vi "DTMF.vi"() -> ()   [LabVIEW 2014]
uses:
  <vilib>/sound2/lvsound2.llb/Sampling Mode.ctl
  <vilib>/sound2/lvsound2.llb/Sound Data Format.ctl
  <vilib>/sound2/lvsound2.llb/Sound Input Read (DBL).vi
  <vilib>/measure/maspectr.llb/FFT Power Spectrum and PSD for N Chan.vi
  <vilib>/measure/NI_MAPro.lvlib
panel:
  in  "Tab Control":enum32{"Info.", "Output", "Details"}(tab)
  in  "Stop":bool
  out "Dialed Number":string
  in  "Number of Samples/ch":i32=5000
  in  "Device ID":u32 format="%.0x"
  out "Raw Data":waveform(dbl)[](graph)
  out "FFT":cluster{"f0":dbl, "df":dbl, "magnitude":dbl[]}[](graph)
  out "Power Spectrum / PSD":cluster{"f0":dbl, "df":dbl, "magnitude":dbl[]}[](array[cluster]) {"magnitude" format="%.2p"; "f0" format="%.2p"; "df" format="%.2p"}
  out "f0":dbl
  out "df":dbl
  out "magnitude":dbl[](array[numeric])
  out "output array":dbl[](array[numeric])
  out "Max":dbl
  out "Coloumn":u32
  out "Raw":u32
  out "Min":dbl
  out "concatenated string":string
  # "This programthe can detect DTMF type sounds and decode them to digits as you know every digits in DTMF modulation contain two tone signal with specified frequency.\nfirst program captures sound from environment and make FFT from that , then the created PSD array processed to retrieve first 2frequency with most power and then realize reffered digit."
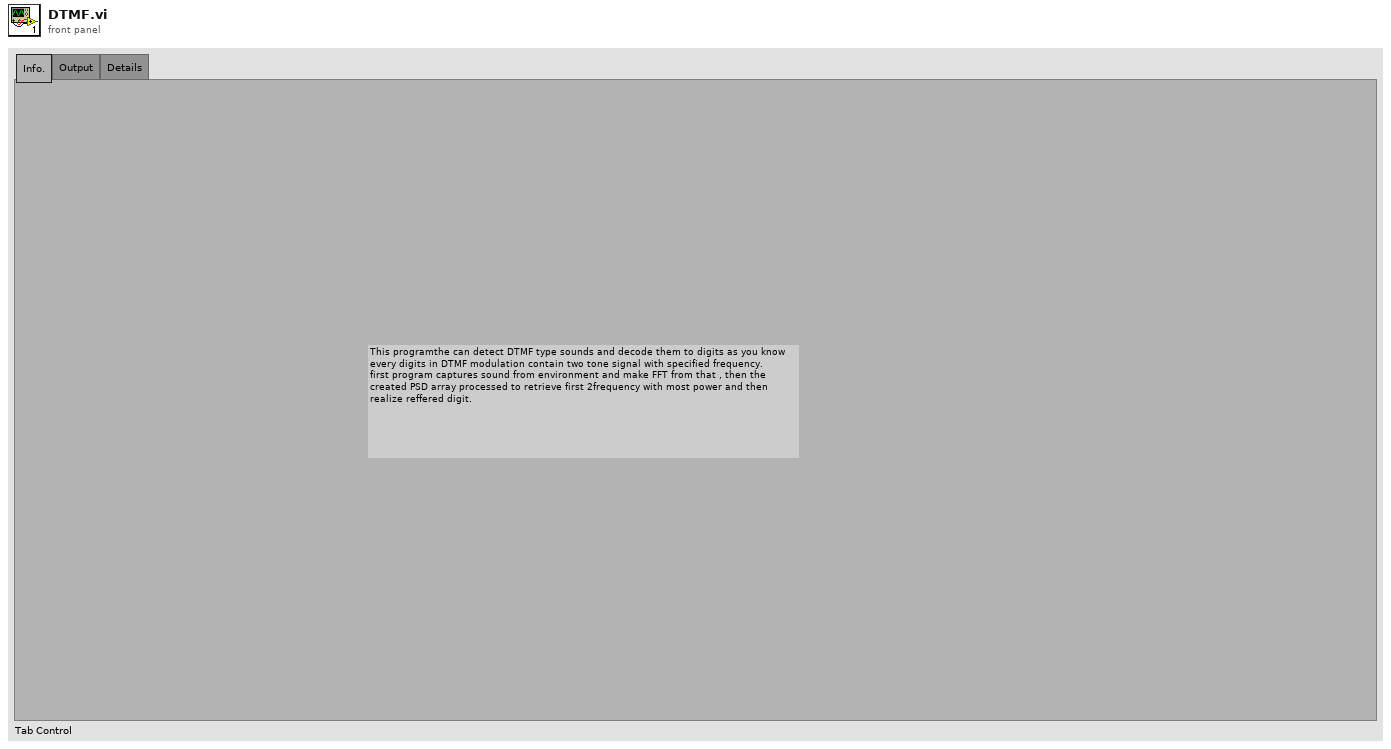
[diagram p1: front panel]
types:
  T1 = typedef "Sound Data Format.ctl" = cluster{"sample rate (S/s)":dbl, "number of channels":i32, "bits per sample":i32}
  T2 = typedef "Sampling Mode.ctl" = i32
  T3 = typedef "Sound Input Task ID.ctl" = u32
  T4 = cluster{"Power Spectrum / PSD[0]":cluster{"f0":dbl, "df":dbl, "magnitude":dbl[]}, "Power Spectrum / PSD[1]":cluster{"f0":dbl, "df":dbl, "magnitude":dbl[]}, "Power Spectrum / PSD[2]":cluster{"f0":dbl, "df":dbl, "magnitude":dbl[]}, "Power Spectrum / PSD[3]":cluster{"f0":dbl, "df":dbl, "magnitude":dbl[]}, "Power Spectrum / PSD[4]":cluster{"f0":dbl, "df":dbl, "magnitude":dbl[]}, "Power Spectrum / PSD[5]":cluster{"f0":dbl, "df":dbl, "magnitude":dbl[]}, "Power Spectrum / PSD[6]":cluster{"f0":dbl, "df":dbl, "magnitude":dbl[]}, "Power Spectrum / PSD[7]":cluster{"f0":dbl, "df":dbl, "magnitude":dbl[]}, "Power Spectrum / PSD[8]":cluster{"f0":dbl, "df":dbl, "magnitude":dbl[]}}
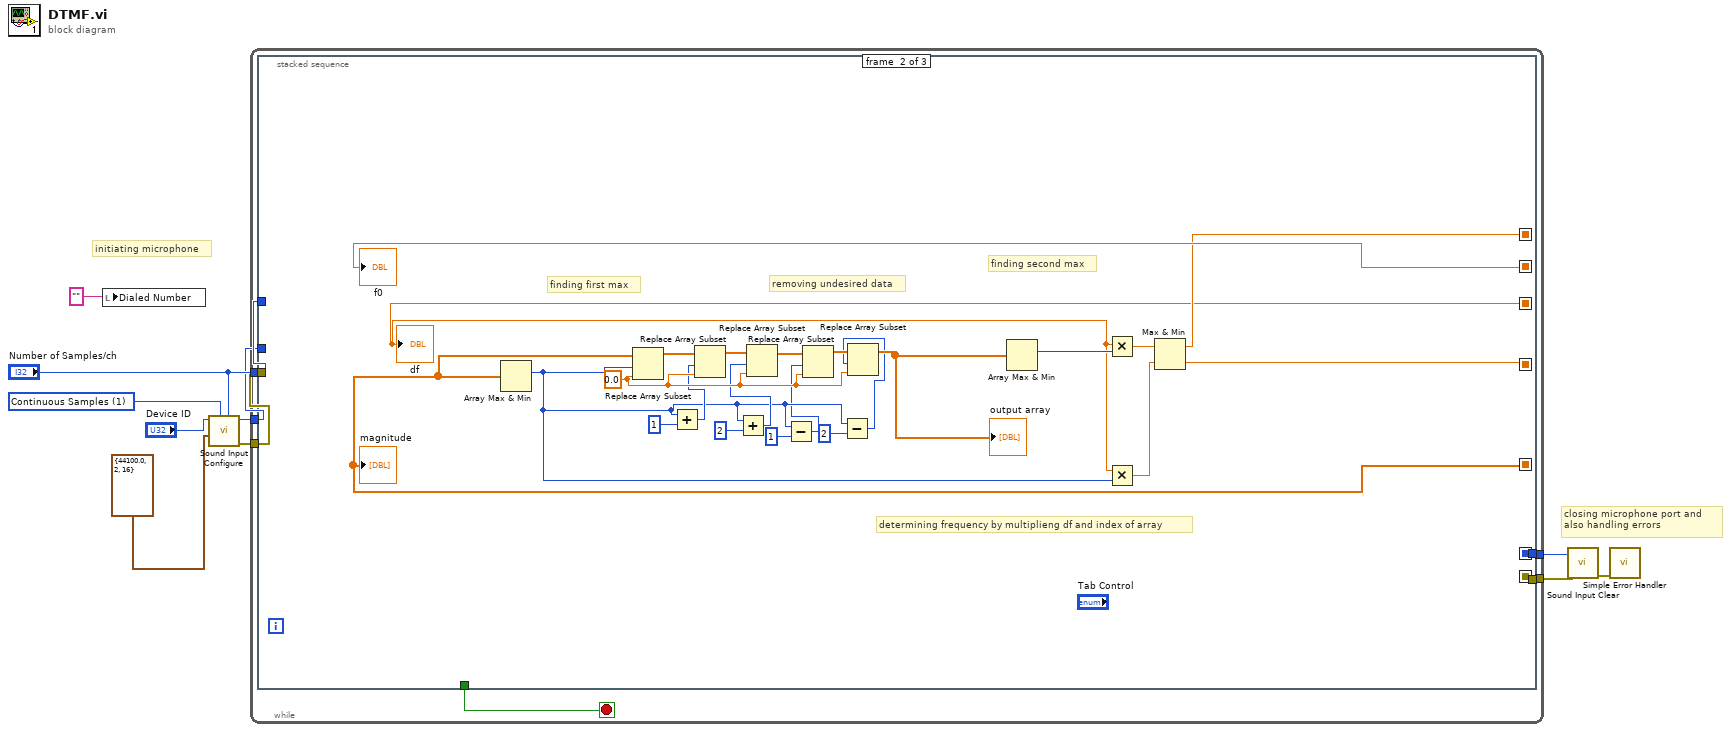
[diagram p0: block diagram]
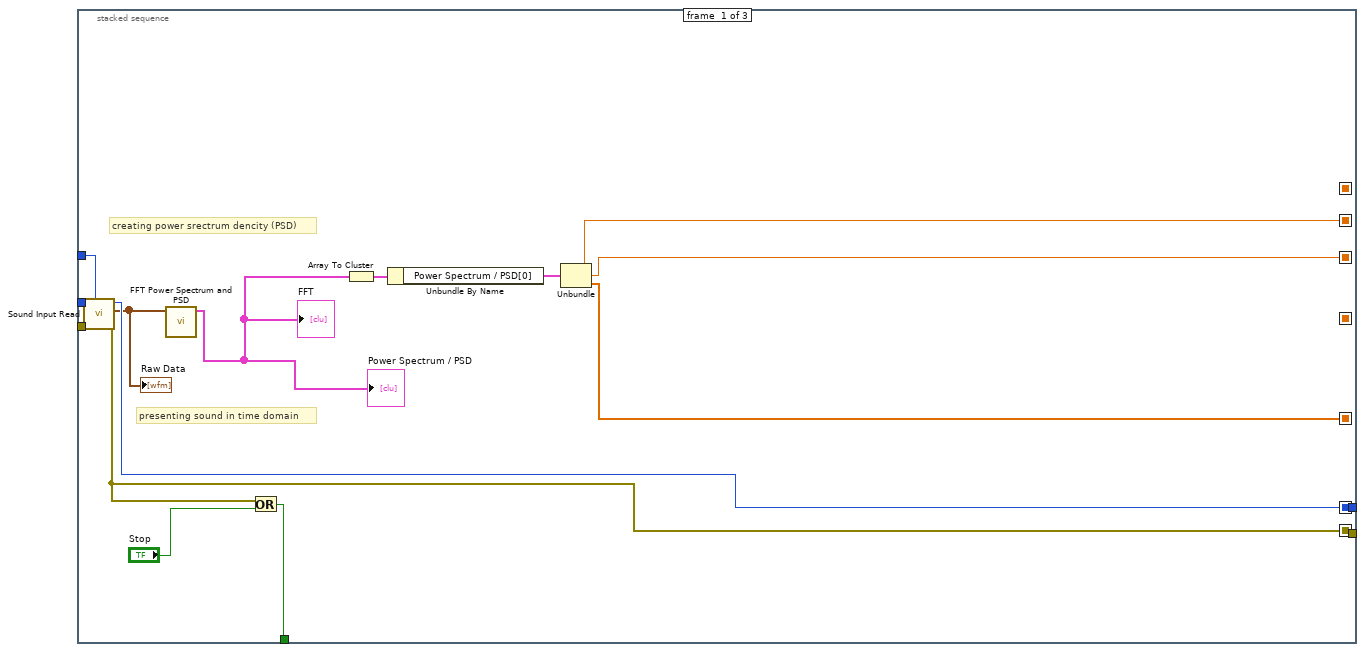
[diagram p2: hidden frame]
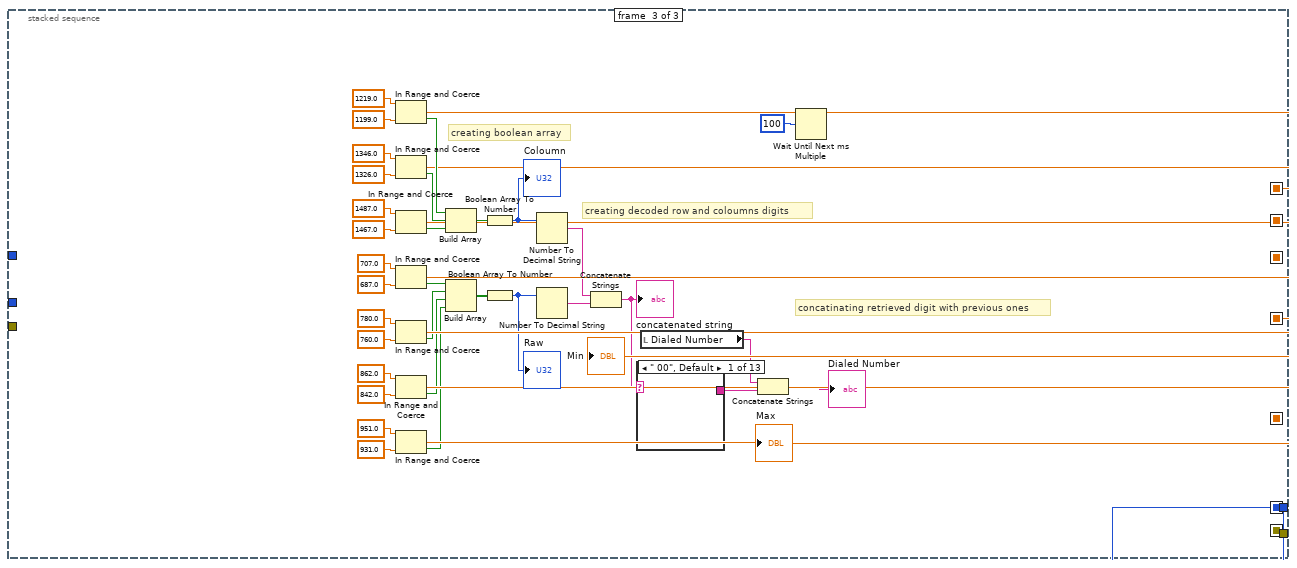
[diagram p3: hidden frame]
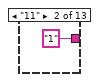
[diagram p4: hidden frame]
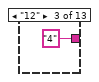
[diagram p5: hidden frame]
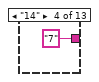
[diagram p6: hidden frame]
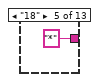
[diagram p7: hidden frame]
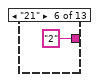
[diagram p8: hidden frame]
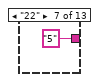
[diagram p9: hidden frame]
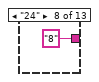
[diagram p10: hidden frame]
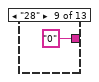
[diagram p11: hidden frame]
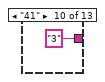
[diagram p12: hidden frame]
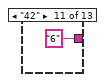
[diagram p13: hidden frame]
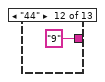
[diagram p14: hidden frame]
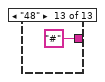
[diagram p15: hidden frame]
diagram:
  w9 = T2 1 items=["Finite Samples", "Continuous Samples"] ("sample mode")
  # "closing microphone port and \nalso handling errors"
  # "initiating microphone"
  n1 = local write "Dialed Number"("") -> ()
  n2 = call <vilib>:"Sound Input Configure.vi"("number of samples/ch"="Number of Samples/ch", "sample mode"=w9, "sound format"=T1 {"sample rate (S/s)"=44100.0, "number of channels"=2, "bits per sample"=16} ("Sound Format"), "device ID"="Device ID") -> ("error out"=w5:errorcluster, "task ID"=w6:T3)  [unwired: 6 in]
  n3 = while {
    tunnel: "Number of Samples/ch" -> [w16]
    tunnel: [w15] -> w1
    tunnel: [w14] -> w2
    tunnel: w6 -> [w13]
    tunnel: w5 -> [w12]
    stop <- w11 stop-if-true
    n4 = stacked-sequence {
      seq-local: [w29 _ _] -> [_ w55 _]
      seq-local: [w28 _ _] -> [_ w54 _]
      seq-local: [w20 _ _] -> [_ w47 _]
      seq-local: [w21 _ _] -> [_ w50 _]
      seq-local: [w19 _ _] -> [_ w31 _]
      seq-local: [_ w55 _] -> [_ _ w91]
      seq-local: [_ w54 _] -> [_ _ w90]
      seq-local: [_ w49 _] -> [_ _ w80]
      seq-local: [_ w48 _] -> [_ _ w78]
      tunnel: w16 -> [w30 _ _]
      tunnel: w13 -> [w27 _ _]
      tunnel: w12 -> [w26 _ _]
      tunnel: [w17 _ _] -> w11
      tunnel: [_ _ w91] -> w15
      tunnel: [_ _ w90] -> w14
      frame #0 {
        # "presenting sound in time domain"
        # "creating power srectrum dencity (PSD)"
        n5 = call-poly <vilib>:"Sound Input Read.vi"("number of samples/ch"=w30, "error in (no error)"=w26, "task ID"=w27) -> ("error out"=w29:errorcluster, "data"=w23:waveform(dbl)[], "task ID out"=w28:T3)  [unwired: 6 in]
        "Raw Data" <- w23
        n6 = call-poly <vilib>:"FFT Power Spectrum and PSD.vi"("time signals"=w23) -> ("Power Spectrum / PSD"=w22:cluster{"f0":dbl, "df":dbl, "magnitude":dbl[]}[])  [unwired: 7 in, 3 out]
        "FFT" <- w22
        "Power Spectrum / PSD" <- w22
        n7 = Or(x=w29, y="Stop") -> (x .or. y?=w17:bool)
        n8 = Array To Cluster(array=w22) -> (cluster=w25:T4)
        n9 = Unbundle By Name(w25) -> ("Power Spectrum / PSD[0]"=w24:cluster{"f0":dbl, "df":dbl, "magnitude":dbl[]})
        n10 = Unbundle(w24) -> ("f0"=w21:dbl, "df"=w20:dbl, "magnitude"=w19:dbl[])
      }
      frame #1 {
        w41 = 0.0 ("new element/subarray")
        # "removing undesired data"
        # "determining frequency by multiplieng df and index of array"
        # "finding second max"
        # "finding first max"
        n11 = Array Max & Min(array=w31) -> (max index (indices)=w34:i32)  [unwired: 3 out]
        n12 = Replace Array Subset(array=w31, new element=w41, index=w34) -> (w42:dbl[])
        n13 = Add(x=w34, y=1) -> (x+y=w39:i32)
        n14 = Replace Array Subset(array=w42, new element=w41, index=w39) -> (w43:dbl[])
        n15 = Add(x=w34, y=2) -> (x+y=w37:i32)
        n16 = Replace Array Subset(array=w43, new element=w41, index=w37) -> (w44:dbl[])
        n17 = Subtract(x=w34, y=1) -> (x-y=w32:i32)
        n18 = Replace Array Subset(array=w44, new element=w41, index=w32) -> (w45:dbl[])
        n19 = Subtract(x=w34, y=2) -> (x-y=w33:i32)
        n20 = Replace Array Subset(array=w45, new element=w41, index=w33) -> (w46:dbl[])
        "output array" <- w46
        n21 = Array Max & Min(array=w46) -> (max index (indices)=w51:i32)  [unwired: 3 out]
        n22 = Multiply(x=w47, y=w51) -> (x*y=w52:dbl)
        n23 = Multiply(x=w47, y=w34) -> (x*y=w53:dbl)
        n24 = Max & Min(x=w52, y=w53) -> (max(x,y)=w49:dbl, min(x,y)=w48:dbl)
        "f0" <- w50
        "df" <- w47
        "magnitude" <- w31
      }
      frame #2 {
        # "creating decoded row and coloumns digits"
        # "creating boolean array"
        # "concatinating retrieved digit with previous ones"
        n25 = In Range and Coerce(upper limit=1219.0, x=w80, lower limit=1199.0) -> (In Range?=w89:bool)  [unwired: 1 out]
        n26 = In Range and Coerce(upper limit=1346.0, x=w80, lower limit=1326.0) -> (In Range?=w88:bool)  [unwired: 1 out]
        n27 = In Range and Coerce(upper limit=1487.0, x=w80, lower limit=1467.0) -> (In Range?=w87:bool)  [unwired: 1 out]
        n28 = In Range and Coerce(upper limit=707.0, x=w78, lower limit=687.0) -> (In Range?=w69:bool)  [unwired: 1 out]
        n29 = In Range and Coerce(upper limit=780.0, x=w78, lower limit=760.0) -> (In Range?=w68:bool)  [unwired: 1 out]
        n30 = In Range and Coerce(upper limit=862.0, x=w78, lower limit=842.0) -> (In Range?=w67:bool)  [unwired: 1 out]
        n31 = In Range and Coerce(upper limit=951.0, x=w78, lower limit=931.0) -> (In Range?=w66:bool)  [unwired: 1 out]
        n32 = Build Array(w89, w88, w87) -> (w79:bool[])
        n33 = Build Array(w69, w68, w67, w66) -> (w65:bool[])
        n34 = Boolean Array To Number(Boolean array=w79) -> (number=w61:u32)
        "Coloumn" <- w61
        n35 = Boolean Array To Number(Boolean array=w65) -> (number=w60:u32)
        "Raw" <- w60
        n36 = Number To Decimal String(number=w61) -> (decimal integer string=w63:string)  [unwired: 1 in]
        n37 = Number To Decimal String(number=w60) -> (decimal integer string=w62:string)  [unwired: 1 in]
        n38 = Concatenate Strings(w63, w62) -> (w64:string)
        "concatenated string" <- w64
        n39 = case shown="\" 00\", Default" w64 {
          tunnel: [_ "1" "4" "7" "*" "2" "5" "8" "0" "3" "6" "9" "#"] -> w59
          frame " 00", Default {
          }
          frame "11" {
          }
          frame "12" {
          }
          frame "14" {
          }
          frame "18" {
          }
          frame "21" {
          }
          frame "22" {
          }
          frame "24" {
          }
          frame "28" {
          }
          frame "41" {
          }
          frame "42" {
          }
          frame "44" {
          }
          frame "48" {
          }
        }
        n40 = local read "Dialed Number"() -> (w57:string)
        n41 = Concatenate Strings(w57, w59) -> (→"Dialed Number":string)
        n42 = Wait Until Next ms Multiple(millisecond multiple=u32 100) -> ()  [unwired: 1 out]
        "Max" <- w80
        "Min" <- w78
      }
    }
  }
  n43 = call <vilib>:"Sound Input Clear.vi"("error in (no error)"=w1, "task ID"=w2) -> ("error out"=w4:errorcluster)  [unwired: 9 in]
  n44 = call <vilib>:"Simple Error Handler.vi"("error in (no error)"=w4) -> ()  [unwired: 4 in, 5 out]
